vi "Vision Processing2.vi"(11 "Image Size":T1=enum."320x240") -> ()   [LabVIEW 2014]
uses:
  Vision Support Code/Camera Types.ctl
  <vilib>/Rock Robotics/WPI/Camera/WPI_CameraImageSize.ctl
  <vilib>/Rock Robotics/WPI/Camera/WPI_CameraWhite Balance Values.ctl
  <vilib>/Rock Robotics/WPI/Camera/WPI_CameraExposure Values.ctl
  <vilib>/Rock Robotics/WPI/Camera/WPI_CameraFrameRate.ctl
  <vilib>/vision/NI_Vision_Development_Module.lvlib
panel:
  in  "Camera Type":T2=enum."MS HD3000 square"
  in  "Image Path":path=path "Sample Images/KicoffFilmingVision"
  in  "image files":string[](array[string])
  in  "Aspect Fudge Factor":dbl=1.0
  out "Detected Totes":T3(array[cluster]) {"Normalized Rect"."Numeric 5" format="%#_2g"; "Normalized Rect"."Numeric 3" format="%#_2g"; "Normalized Rect"."Numeric 2" format="%#_2g"; "Normalized Rect"."Numeric" format="%#_2g"}
  in  "Score Threshold":dbl=75.0
  in  "Source":enum32{"Files", "Camera"}(tab)
  in  "Images":i32(listbox)
  in  "Folder Location":path=path "Sample Images/KicoffFilmingVision"
  in  "Annotate":bool=TRUE
  out "ms to process":u32
  out "Sorted Scores":T4(array[cluster]) {"Aspect Ratio" format="%#_3g"; "Area Score" format="%#_3g"; "X" format="%#_3g"; "Y" format="%#_3g"}
  out "Particles":i32
  in  "Ring Light Color":T5={"Hue"={101.37467765958063, 64.10933859299683}, "Sat"={88.03571428571429, 255.0}, "Val"={133.57142857142858, 255.0}} {"Hue" scale=0.0..255.0 scale format="%#_3g"}
  out "Masked":T6(plugin-control)
  out "Original Image":T6(plugin-control)
  # "Instructions:\nUse Source to select image files from a directory or use a USB or IP camera connected to your laptop.\nUse the Color of a ring light to threshold and build particles. Adjust calibration if needed.\nSmall modifications to the diagram will allow for intensity processing instead of color.\nAnnotations show the rectangle and the scores from top to bottom."
  # "Density Profile"
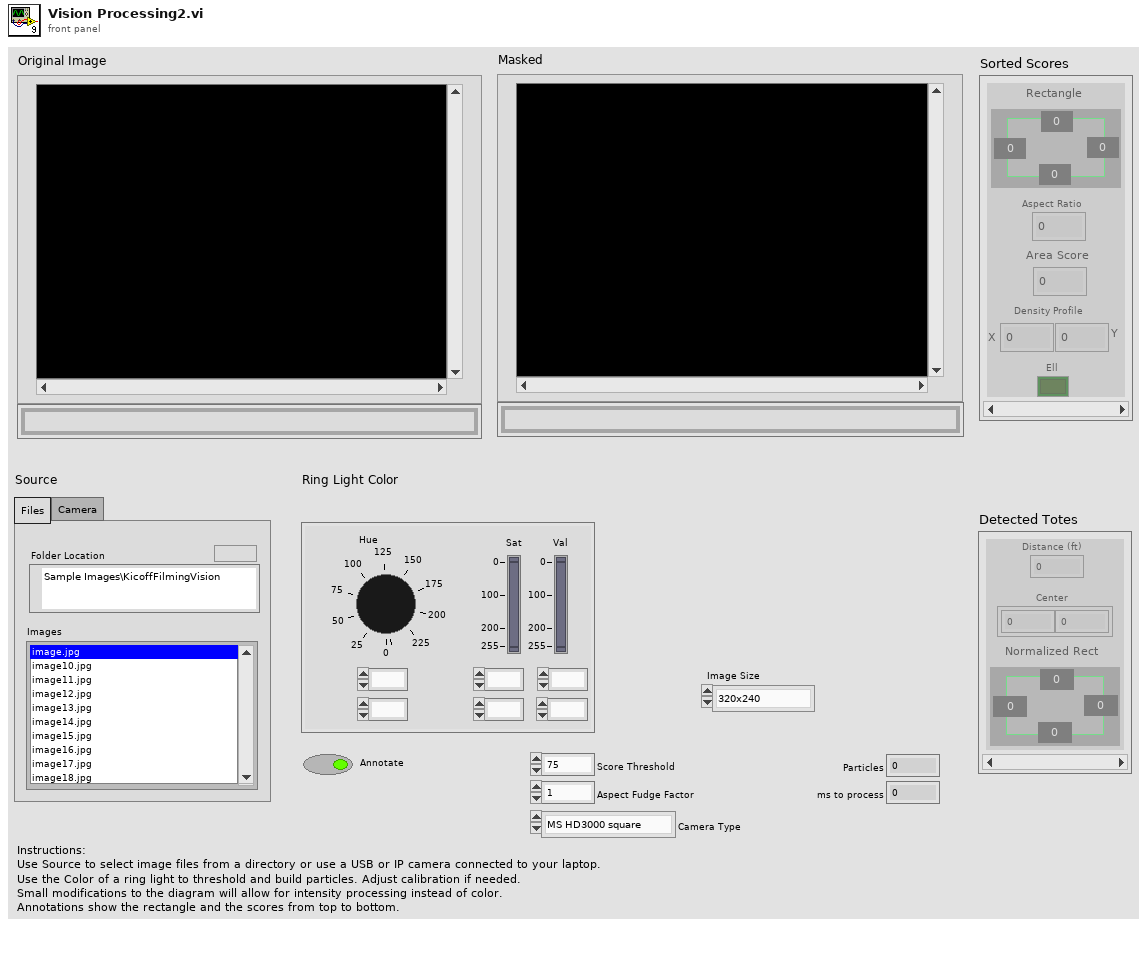
[diagram p1: front panel]
types:
  T1 = typedef "WPI_CameraImageSize.ctl" = enum16{"640x480", "320x240", "160x120", "Custom"}
  T2 = typedef "Camera Types.ctl" = enum16{"206", "1011", "1013", "MS HD3000 square", "MS HD3000 640x480"}
  T3 = cluster{"Distance (ft)":dbl, "Center":cluster{dbl, dbl}, "Normalized Rect":cluster{"Numeric":dbl, "Numeric 2":dbl, "Numeric 3":dbl, "Numeric 5":dbl}}[]
  T4 = cluster{"Rectangle":cluster{"Numeric":dbl, "Numeric 2":dbl, "Numeric 3":dbl, "Numeric 5":dbl}, "Aspect Ratio":dbl, "Area Score":dbl, "X":dbl, "Y":dbl, "Ell":bool}[]
  T5 = cluster{"Hue":cluster{dbl, dbl}, "Sat":cluster{dbl, dbl}, "Val":cluster{dbl, dbl}}
  T6 = typedef "IMAQ Image.ctl" = refnum<image>
  T7 = typedef "WPI_CameraFrameRate.ctl" = u32
  T8 = typedef "WPI_CameraExposure Values.ctl" = enum16{"Auto", "Flicker-free 50 Hz", "Flicker-free 60 Hz", "Hold current", "Custom"}
  T9 = typedef "WPI_CameraWhite Balance Values.ctl" = enum16{"Auto", "Fixed indoor", "Fixed outdoor 1", "Fixed outdoor 2", "Fixed fluorescent 1", "Fixed fluorescent 2", "Hold current", "Custom"}
  T10 = typedef "Particle Parameters" = i32
  T11 = typedef "Image Type" = u32
  T12 = typedef "WPI_CameraDevRef.ctl" = cluster{"Camera Address":string, "CameraStatus":errorcluster}
  T13 = cluster{"Bounding box":cluster{"left":dbl, "top":dbl, "right":dbl, "bottom":dbl}, "Aspect Ratio":dbl, "Area Score":dbl, "X Mask":dbl, "Y Mask":dbl, "Ell":bool}[]
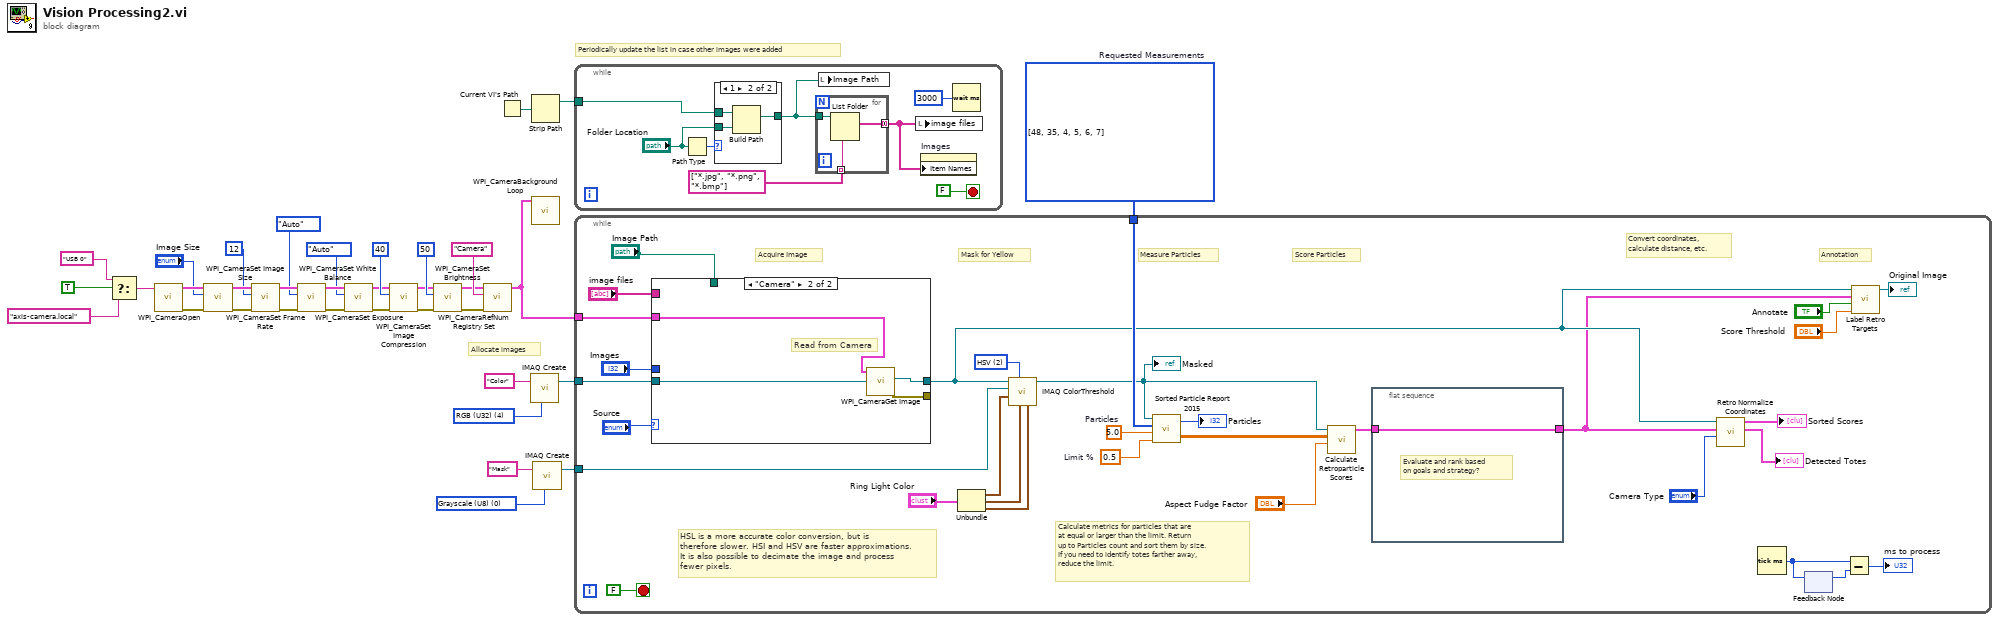
[diagram p0: block diagram]
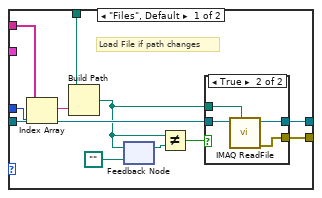
[diagram p3: hidden frame]
diagram:
  w29 = T10[] [48, 35, 4, 5, 6, 7] items=["Center of Mass X", "Center of Mass Y", "First Pixel X", "First Pixel Y", "Bounding Rect Left", "Bounding Rect Top", "Bounding Rect Right", "Bounding Rect Bottom", "Max Feret Diameter Start X", "Max Feret Diameter Start Y", "Max Feret Diameter End X", "Max Feret Diameter End Y", "Max Horiz. Segment Length Left", "Max Horiz. Segment Length Right", "Max Horiz. Segment Length Row", "-", "Bounding Rect Width", "Bounding Rect Height", "Bounding Rect Diagonal", "Perimeter", "Convex Hull Perimeter", "Holes' Perimeter", "Max Feret Diameter", "Equivalent Ellipse Major Axis", "Equivalent Ellipse Minor Axis", "Equivalent Ellipse Minor Axis (Feret)", "Equivalent Rect Long Side", "Equivalent Rect Short Side", "Equivalent Rect Diagonal", "Equivalent Rect Short Side (Feret)", "Average Horiz. Segment Length", "Average Vert. Segment Length", "Hydraulic Radius", "Waddel Disk Diameter", "-", "Area", "Holes' Area", "Particle & Holes' Area", "Convex Hull Area", "Image Area", "-", "Number of Holes", "Number of Horiz. Segments", "Number of Vert. Segments", "-", "Orientation", "Max Feret Diameter Orientation", "-", "% Area/Image Area", "% Area/(Particle & Holes' Area)", "Ratio of Equivalent Ellipse Axes", "Ratio of Equivalent Rect Sides", "-", "Elongation Factor", "Compactness Factor", "Heywood Circularity Factor", "Type Factor", "-", "Sum X", "Sum Y", "Sum XX", "Sum XY", "Sum YY", "Sum XXX", "Sum XXY", "Sum XYY", "Sum YYY", "-", "Moment of Inertia XX", "Moment of Inertia XY", "Moment of Inertia YY", "Moment of Inertia XXX", "Moment of Inertia XXY", "Moment of Inertia XYY", "Moment of Inertia YYY", "Norm. Moment of Inertia XX", "Norm. Moment of Inertia XY", "Norm. Moment of Inertia YY", "Norm. Moment of Inertia XXX", "Norm. Moment of Inertia XXY", "Norm. Moment of Inertia XYY", "Norm. Moment of Inertia YYY", "Hu Moment 1", "Hu Moment 2", "Hu Moment 3", "Hu Moment 4", "Hu Moment 5", "Hu Moment 6", "Hu Moment 7"]  # Requested Measurements
  w32 = T11 0 items=["Grayscale (U8)", "Grayscale (I16)", "Grayscale (SGL)", "Complex (CSG)", "RGB (U32)", "HSL (U32)", "RGB (U64)", "Grayscale (U16)"] ("Image Type")
  w34 = T11 4 items=["Grayscale (U8)", "Grayscale (I16)", "Grayscale (SGL)", "Complex (CSG)", "RGB (U32)", "HSL (U32)", "RGB (U64)", "Grayscale (U16)"] ("Image Type")
  # "Periodically update the list in case other images were added"
  # "Allocate images"
  n1 = Select(t="USB 0" ("format string"), s=TRUE ("dot notation? (F)"), f="axis-camera.local" ("format string")) -> (s? t:f=w3:string)
  n2 = call <vilib>:"WPI_CameraOpen.vi"("Camera Address"=w3) -> ("error out"=w17:errorcluster, "CameraDevRef"=w18:T12)  [unwired: 1 in, 8 out]
  n3 = call <vilib>:"WPI_CameraSet Image Size.vi"("error in (no error)"=w17, "Image Size"="Image Size", "CameraDevRef"=w18) -> ("error out"=w16:errorcluster, "CameraDevRef Out"=w19:T12)  [unwired: 1 in, 6 out]
  n4 = call <vilib>:"WPI_CameraSet Frame Rate.vi"("error in (no error)"=w16, "Frame Rate (fps)"=T7 12, "CameraDevRef"=w19) -> ("error out"=w15:errorcluster, "CameraDevRef Out"=w21:T12)  [unwired: 7 out]
  n5 = call <vilib>:"WPI_CameraSet White Balance.vi"("error in (no error)"=w15, "White Balance"=WPI_CameraWhite_Balance_Values."Auto", "CameraDevRef"=w21) -> ("error out"=w14:errorcluster, "CameraDevRef Out"=w20:T12)  [unwired: 1 in, 6 out]
  n6 = call <vilib>:"WPI_CameraSet Exposure.vi"("error in (no error)"=w14, "Exposure"=WPI_CameraExposure_Values."Auto", "CameraDevRef"=w20) -> ("error out"=w13:errorcluster, "CameraDevRef Out"=w23:T12)  [unwired: 1 in, 6 out]
  n7 = call <vilib>:"WPI_CameraSet Image Compression.vi"("error in (no error)"=w13, "Compression"=40, "CameraDevRef"=w23) -> ("error out"=w12:errorcluster, "CameraDevRef Out"=w22:T12)  [unwired: 7 out]
  n8 = call <vilib>:"WPI_CameraSet Brightness.vi"("error in (no error)"=w12, "Brightness"=50, "CameraDevRef"=w22) -> ("error out"=w10:errorcluster, "CameraDevRef Out"=w11:T12)  [unwired: 7 out]
  n9 = call <vilib>:"WPI_CameraRefNum Registry Set.vi"("error in (no error)"=w10, "refnum name"="Camera", "CameraDevRef"=w11) -> ("CameraDevRef"=w2:T12)  [unwired: 8 out]
  n10 = Current VI's Path() -> (path=w28:path)
  n11 = call "IMAQ Create"("Image Name"="Color", "Image Type"=w34) -> ("New Image"=w33:T6)  [unwired: 2 in, 2 out]
  n12 = Strip Path(path=w28) -> (stripped path=w27:path)  [unwired: 1 out]
  n13 = call <vilib>:"WPI_CameraBackground Loop.vi"("CameraDevRef"=w2) -> ()  [unwired: 11 in]
  n14 = call "IMAQ Create"("Image Name"="Mask", "Image Type"=w32) -> ("New Image"=w30:T6)  [unwired: 2 in, 2 out]
  n15 = while {
    tunnel: w27 -> [w37]
    stop <- FALSE stop-if-true
    n16 = Path Type(1:"Folder Location") -> (0:w39:i16)
    n17 = case shown="1" w39 {
      tunnel: "Folder Location" -> [w44 w47]
      tunnel: [w44 w45] -> w36
      tunnel: w37 -> [_ w46]
      frame 0, Default {
      }
      frame 1 {
        n18 = Build Path(base path=w46, name or relative path=w47) -> (appended path=w45:path)
      }
    }
    n19 = for {
      tunnel: [w50] -> w40 mode=concatenating
      tunnel: w36 -> [w49]
      tunnel: string[] ["*.jpg", "*.png", "*.bmp"] -> [w48] mode=indexing
      n20 = List Folder(path=w49, pattern=w48) -> (filenames=w50:string[])  [unwired: 2 in, 3 out]
    }
    n21 = local write "Image Path"(w36) -> ()
    n22 = local write "image files"(w40) -> ()
    n23 = property on="Images" class="LstBox (strict)"("Item Names"=w40) -> ()  [unwired: 2 in, 2 out]
    n24 = Wait (ms)(milliseconds to wait=u32 3000) -> ()  [unwired: 1 out]
  }
  n25 = while {
    tunnel: w33 -> [w81]
    tunnel: w30 -> [w79]
    tunnel: w29 -> [w73]
    tunnel: w2 -> [w51]
    stop <- FALSE stop-if-true
    w70 = 0.5  # Limit %
    w72 = 5.0  # Particles
    w78 = u16 2 items=["RGB", "HSL", "HSV", "HSI"] ("Color Mode")
    # "Calculate metrics for particles that are\nat equal or larger than the limit. Return\nup to Particles count and sort them by size.\nIf you need to identify totes farther away,\nreduce the limit."
    # "Measure Particles"
    # "Convert coordinates,\ncalculate distance, etc."
    # "Annotation"
    # "Score Particles"
    # "Mask for Yellow"
    # "Acquire Image"
    # "HSL is a more accurate color conversion, but is\ntherefore slower. HSI and HSV are faster approximations.\nIt is also possible to decimate the image and process\nfewer pixels."
    n26 = case shown="\"Camera\"" "Source" {
      tunnel: [w93 w100] -> _
      tunnel: [w94 w101] -> w58
      tunnel: w81 -> [w92 w102]
      tunnel: "image files" -> [w84 _]
      tunnel: "Images" -> [w91 _]
      tunnel: "Image Path" -> [w89 _]
      tunnel: w51 -> [_ w103]
      frame "Files", Default {
        # "Load File if path changes"
        n27 = Index Array(array=w84, index=w91) -> (element=w90:string)
        n28 = Build Path(base path=w89, name or relative path=w90) -> (appended path=w85:path)
        n29 = feedback-in #1(w85) -> ()
        n30 = feedback #1(path "" ("appended path")) -> (w87:path)
        n31 = Not Equal?(x=w85, y=w87) -> (x != y?=w88:bool)
        n32 = case shown="True" w88 {
          tunnel: [w95 w99] -> w94
          tunnel: [_ w98] -> w93
          tunnel: w92 -> [w95 w97]
          tunnel: w85 -> [_ w96]
          frame False {
          }
          frame True {
            n33 = call "IMAQ ReadFile"("File Path"=w96, "Image"=w97) -> ("error out"=w98:errorcluster, "Image Out"=w99:T6)  [unwired: 5 in, 3 out]
          }
        }
      }
      frame "Camera" {
        # "Read from Camera"
        n34 = call <vilib>:"WPI_CameraGet Image.vi"("Image"=w102, "CameraDevRef"=w103) -> ("error out"=w100:errorcluster, "Image Out"=w101:T6)  [unwired: 7 in, 1 out]
      }
    }
    n35 = Unbundle("Ring Light Color") -> ("Hue"=w77:cluster{dbl, dbl}, "Sat"=w76:cluster{dbl, dbl}, "Val"=w75:cluster{dbl, dbl})
    n36 = call "IMAQ ColorThreshold"("Blue or Luma or Val or Inten Range"=w75, "Green or Sat Range"=w76, "Color Mode"=w78, "Red or Hue Range"=w77, "Image Dst"=w79, "Image Src"=w58) -> ("Image Dst Out"=w63:T6)  [unwired: 4 in, 1 out]
    "Masked" <- w63
    n37 = call "Sorted Particle Report 2015.vi"("Min Area Size %"=w70, "Particle Count Limit"=w72, "Pixel Measurements"=w73, "Image in"=w63) -> ("Sorted Data"=w60:dbl[][], "Particles"=→"Particles":i32)
    n38 = call "Calculate Retroparticle Scores.vi"("Aspect Fudge Factor"="Aspect Fudge Factor", "Sorted Data"=w60, "Image in"=w63) -> ("Scores"=w62:T13)  [unwired: 8 in]
    n39 = flat-sequence {
      tunnel: w62 -> [w83]
      tunnel: [w83] -> w55
      frame #0 {
        # "Evaluate and rank based\non goals and strategy?"
      }
    }
    n40 = call "Retro Normalize Coordinates.vi"("Camera Type"="Camera Type", "Scores"=w55, "Image in"=w58) -> ("Found Totes"=→"Detected Totes":T3, "Sorted Scores"=→"Sorted Scores":T4)  [unwired: 7 in]
    n41 = Tick Count (ms)() -> (millisecond timer value=w68:u32)
    n42 = feedback-in #2(w68) -> ()
    n43 = feedback #2() -> (w69:u32)  [unwired: 1 in]
    n44 = Subtract(x=w68, y=w69) -> (x-y=→"ms to process":u32)
    n45 = call "Label Retro Targets.vi"("Score Threshold"="Score Threshold", "Annotate"="Annotate", "Scores"=w55, "Image in"=w58) -> ("Image out"=→"Original Image":T6)  [unwired: 7 in]
  }
